vi "(SubVI)Scope_Start.vi"(7 "Mode":T1, 8 "error in (no error)":errorcluster caption="에러 입력(에러 없음)", 11 "Recording Time":u16) -> (0 "error out":errorcluster caption="에러 출력")   [LabVIEW 2020]
uses:
  Controls/(Ctrl)Scope_Mode.ctl
  Variables/(Var)System Variables.vi
  Serial/Instance VIs/(SubVI)Serial_Write.vi
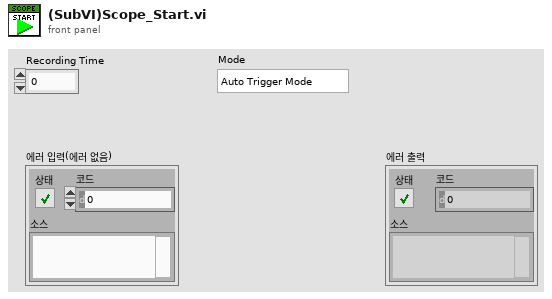
[diagram p1: front panel]
types:
  T1 = typedef "(Ctrl)Scope_Mode.ctl" = enum8{"Auto Trigger Mode", "Continuous Mode"}
  T2 = typedef "Haptic IC.lvclass/(Ctrl)IC Type.ctl" = enum8{"DW7800", "DW7802", "DW7912", "DW7914"}
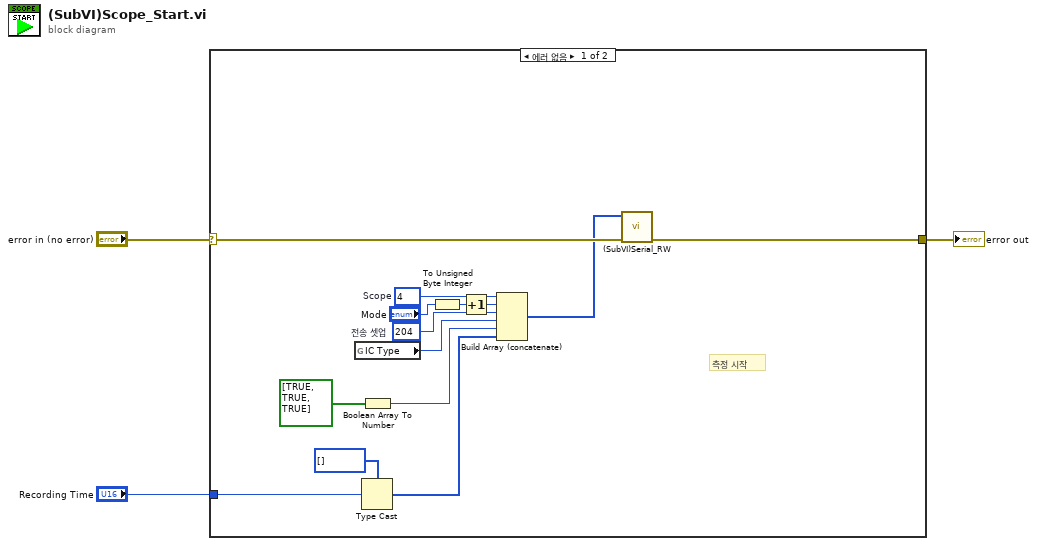
[diagram p0: block diagram]
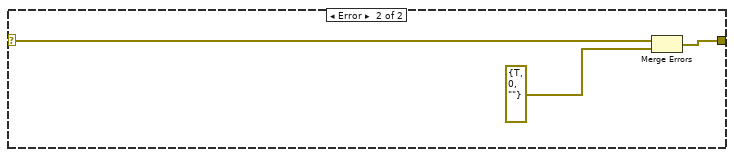
[diagram p2: hidden frame]
diagram:
  n1 = case shown="에러 없음" "error in (no error)" {
    selector: "error in (no error)" -> [w14 w20]
    tunnel: [w5 w19] -> w3
    tunnel: "Recording Time" -> [w8 _]
    frame No Error {
      w15 = u8 204  # 전송 셋업
      w17 = u8 4  # Scope
      # "측정 시작"
      n2 = global read "(Var)System Variables.vi" "IC Type"() -> (w10:T2)
      n3 = Type Cast(type=u8[] [] ("타입"), x=w8) -> (*(type *) &x=w6:u8[])
      n4 = Boolean Array To Number ("불리언 배열을 숫자로")(Boolean array=bool[] [TRUE, TRUE, TRUE] ("Activated Ch")) -> (number=w9:u8)
      n5 = To Unsigned Byte Integer(number="Mode") -> (unsigned 8bit integer=w12:u8)
      n6 = Increment(x=w12) -> (x+1=w11:u8)
      n7 = Build Array (concatenate)(w17, w11, w15, w10, w9, w6) -> (w13:u8[])
      n8 = call-poly "(SubVI)Serial_RW.vi"("error in (no error)"=w14, "Data to Write"=w13) -> ("error out"=w5:errorcluster)  [unwired: 9 in]
    }
    frame Error {
      n9 = Merge Errors(w20, errorcluster {"status"=TRUE, "code"=0, "source"=""} ("에러 입력")) -> (w19:errorcluster)
    }
  }
  "error out" <- w3
